vi "Set Server gRPC UEs.vi"(10 "Server RPC Methods":T1, 11 "OOP Server in":refnum<class "MeasurementService_Template.lvclass">) -> (3 "OOP Server out":refnum<class "MeasurementService_Template.lvclass">)   [LabVIEW 2020, in "LineRegulation.lvlib" / "MeasurementService_Template.lvclass"]
uses:
  MeasurementService_Template.lvclass
  typeDefs/Server gRPC UEs.ctl
  <vilib>/gRPC/LabVIEW gRPC Library/Server API/typeDefs/gRPCId Cluster.ctl
  <vilib>/gRPC/LabVIEW gRPC Library/Server API/typeDefs/grpcId.ctl
  MeasurementService_Template.lvclass/MeasurementService_Template.ctl
  <vilib>/gRPC/LabVIEW gRPC Library/gprc-lvsupport-release.lvlib
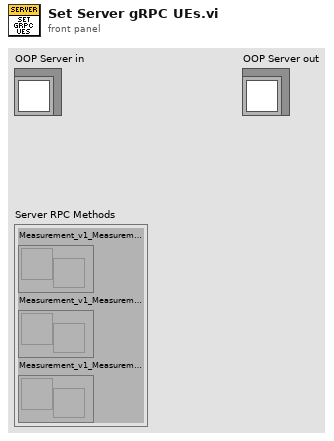
[diagram p1: front panel]
types:
  T1 = typedef "LineRegulation.lvlib/MeasurementService_Template.lvclass/Server gRPC UEs.ctl" = cluster{"Measurement_v1_MeasurementService_GetMetadata gRPC UE":refnum<user-event>, "Measurement_v1_MeasurementService_Measure gRPC UE":refnum<user-event>, "Measurement_v1_MeasurementService_StopService gRPC UE":refnum<user-event>}
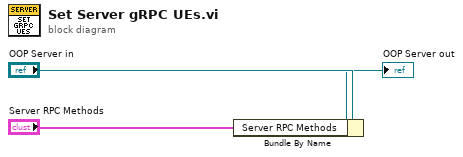
[diagram p0: block diagram]
diagram:
  n1 = Bundle By Name(cluster="OOP Server in", "Server RPC Methods"="Server RPC Methods") -> (→"OOP Server out":refnum<class "MeasurementService_Template.lvclass">)
